vi "Forward Kinematics.vi"(0 "theta":dbl[](array[numeric])=[0.0, 0.0, 0.0] format="%#_15g", 1 "v1d":dbl[](array[numeric]), 2 "v2d":dbl[](array[numeric]), 3 "v3d":dbl[](array[numeric]), 5 "alpha1":dbl=1.5707963267948966, 7 "alpha2":dbl=1.5707963267948966, 9 "beta1":dbl=0.816496580927726, 11 "gamma2":dbl=1.2566370614359172) -> (4 "v1":dbl[](array[numeric]), 6 "v2":dbl[](array[numeric]), 8 "v3":dbl[](array[numeric]), 10 "error?":bool=TRUE, 15 "message":string="Error -23024 occurred at an unidentified location\r\n\r\nPossible reason(s):\n\r\nAnalysis:  No root found.")   [LabVIEW 2017]
uses:
  <vilib>/Utility/error.llb/DialogType.ctl
  <vilib>/Analysis/_algsub.llb/Real Vector Norm.vi
  <vilib>/gmath/zero.llb/nD Nonlinear System Single Solution (Formula).vi
  <vilib>/gmath/NI_Gmath.lvlib
  <vilib>/Analysis/NI_AALPro.lvlib
panel:
  out "beta2":dbl=0.7460127831658564
  out "F(X)":string[](array[string])=["a*d + b*e + c*f - cos(1.256637)", "d*g + e*h + f*i - cos(1.256637)", "g*a + h*b + i*c - cos(1.256637)", "(1.000000)*a + (-0.000000)*b + (-0.000000)*c - cos(1.570796)", "(-0.500000)*d + (0.866025)*e + (-0.000000)*f - cos(1.570796)", "(-0.500000)*g + (-0.866025)*h + (-0.000000)*i - cos(1.570796)", "a^2 + b^2 + c^2 - 1", "d^2 + e^2 + f^2 - 1", "g^2 + h^2 + i^2 - 1"]
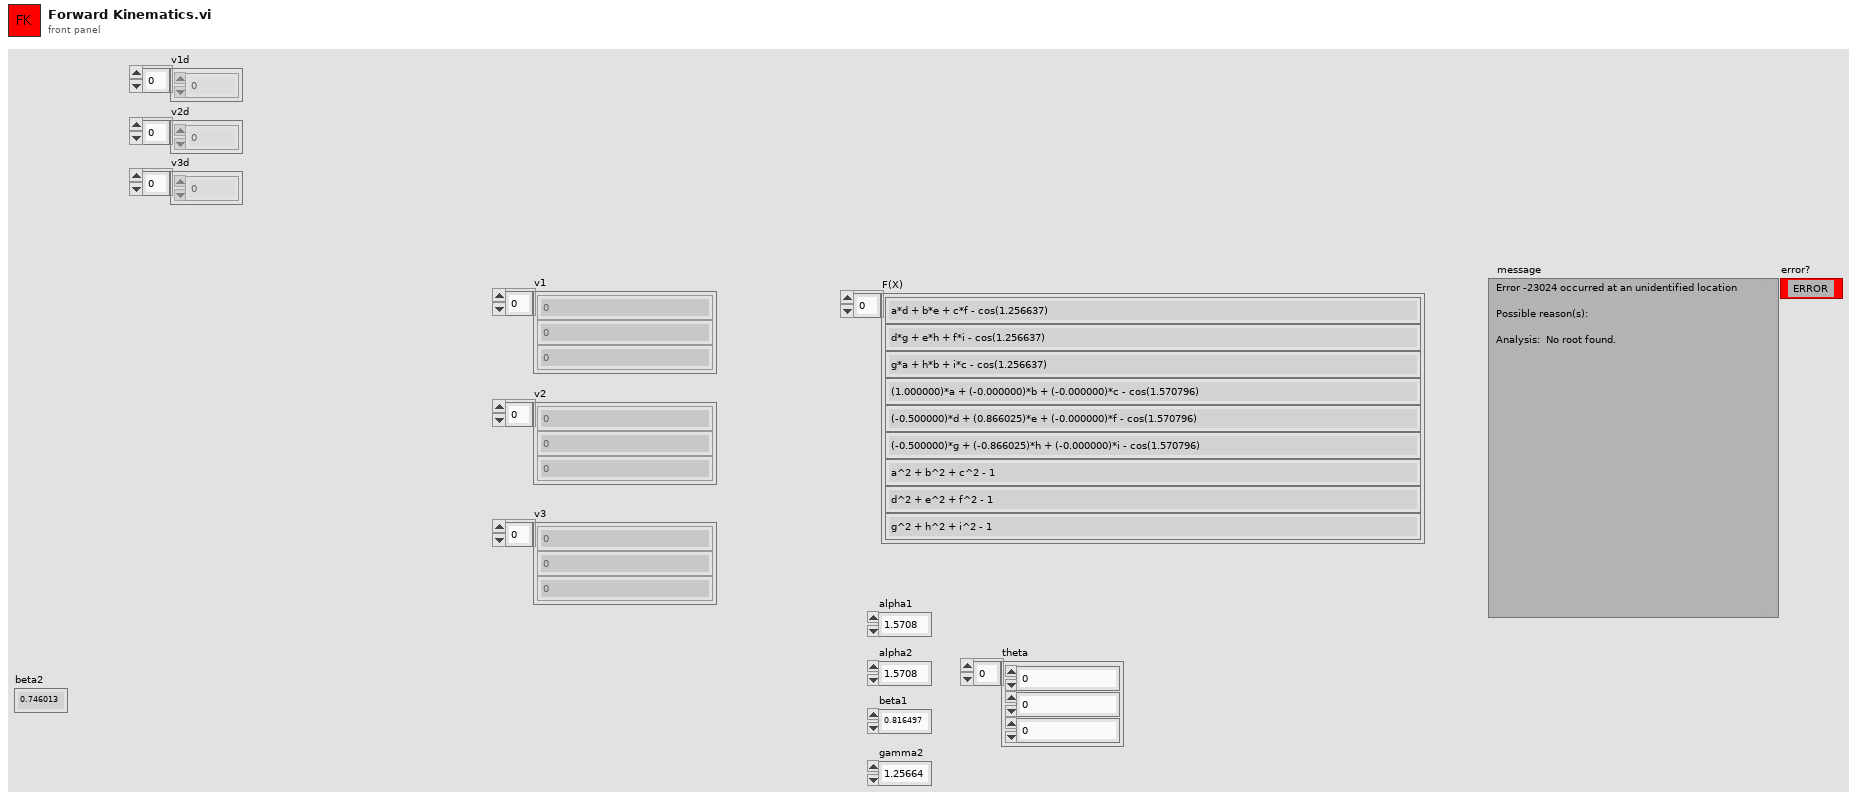
[diagram p1: front panel]
types:
  T1 = typedef "DialogType.ctl" = u16
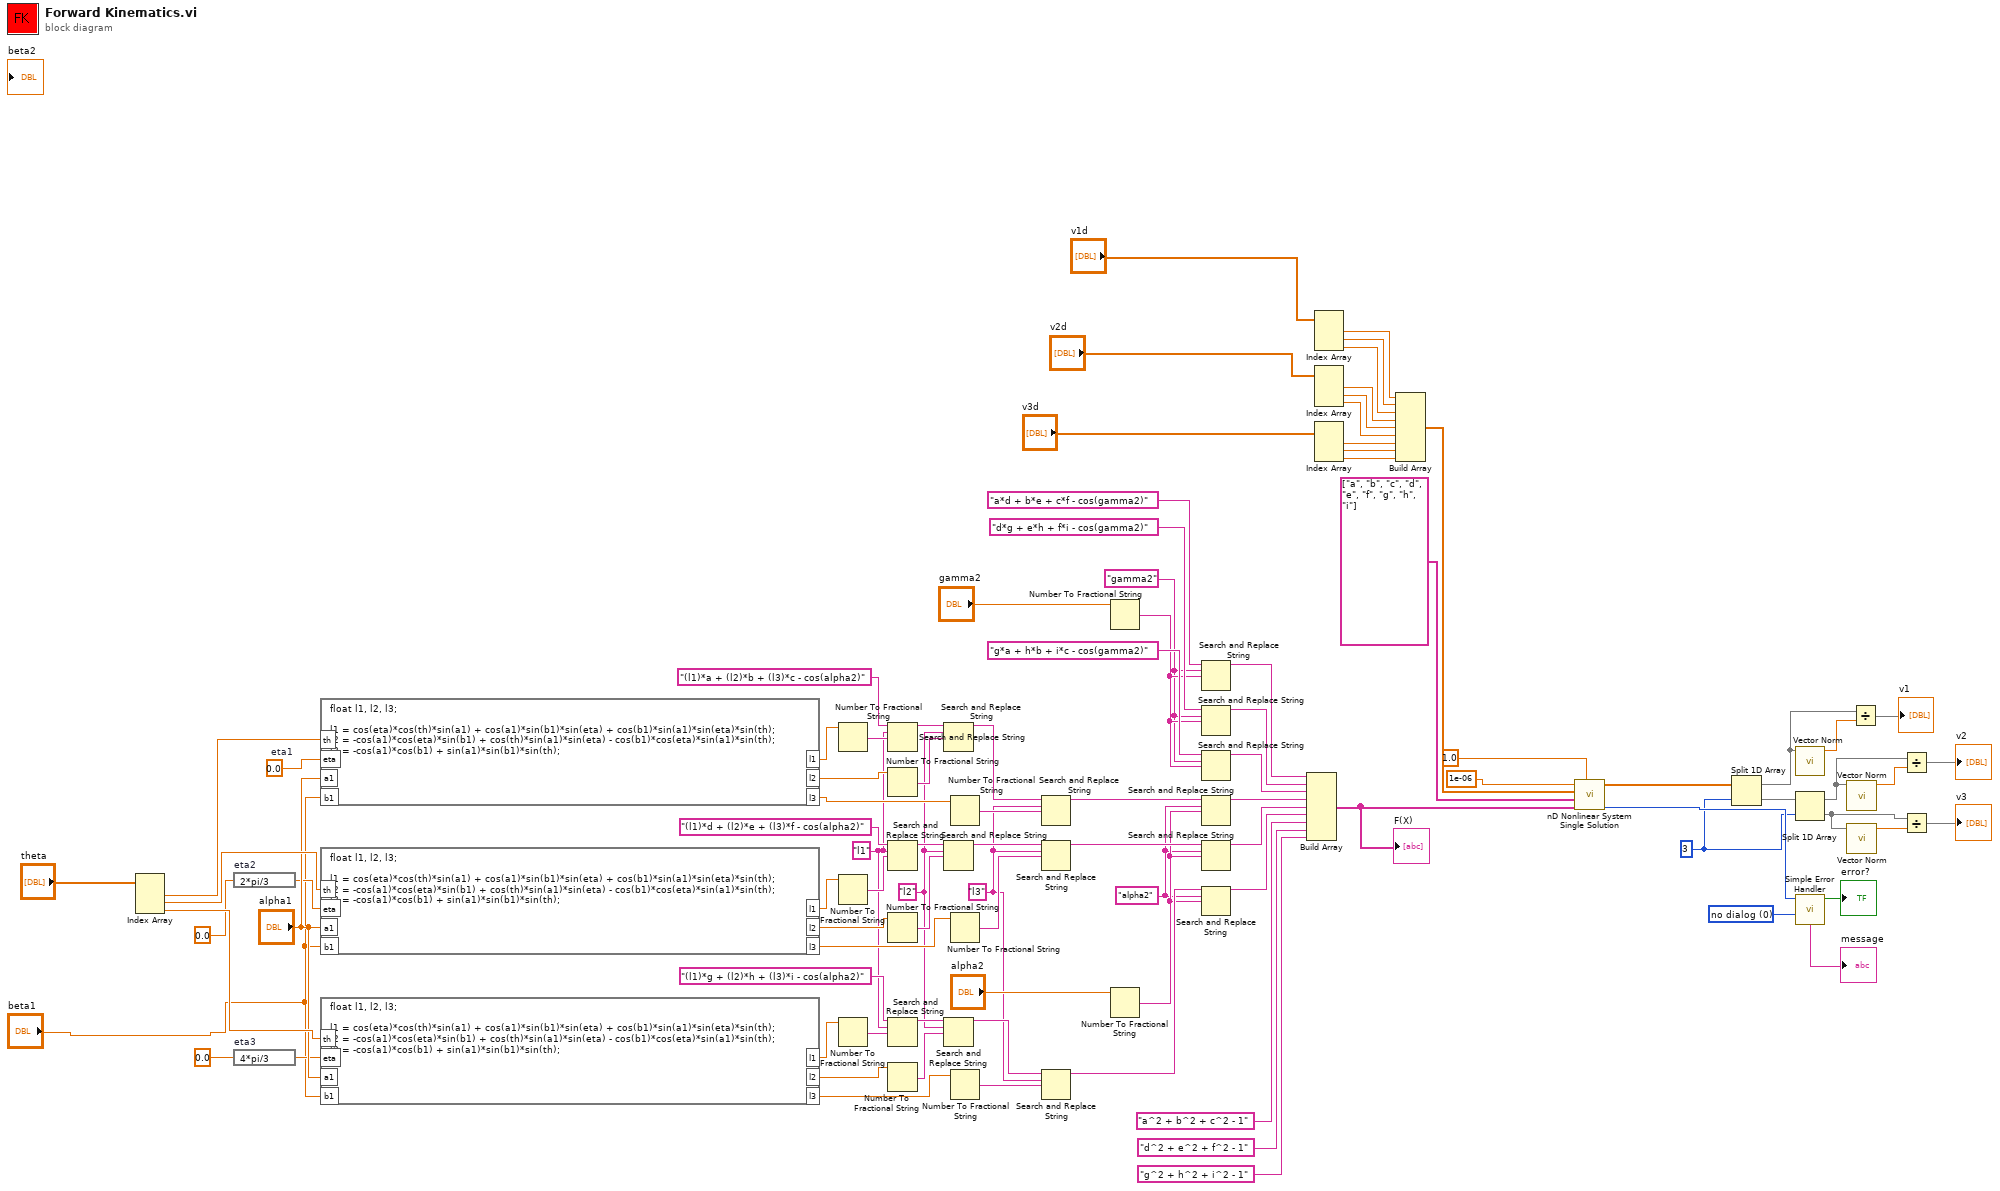
[diagram p0: block diagram]
diagram:
  w21 = 3 ("index")
  w26 = T1 0 items=["no dialog", "OK message", "continue or stop message", "OK message + warnings", "continue/stop + warnings"] ("type of dialog (OK msg:1)")
  w40 = "alpha2" ("search string")
  w41 = "l3" ("search string")
  w42 = "l2" ("search string")
  w43 = "l1" ("search string")
  w39 = "gamma2" ("replace string (\"\")")
  w93 = 0.0  # eta1
  n1 = Index Array(array="theta") -> (element #1=w94:dbl, element #2=w61:dbl, element #3=w60:dbl)  [unwired: 3 in]
  n2 = expression code="2*pi/3" "eta2"(0.0) -> (w52:dbl)
  n3 = expression code="4*pi/3" "eta3"(0.0) -> (w50:dbl)
  n4 = formula code="float l1, l2, l3;\n\nl1 = cos(eta)*cos(th)*sin(a1) + cos(a1)*sin(b1)*sin(eta) + cos(b1)*sin(a1)*sin(eta)*sin(th);\nl2 = -cos(a1)*cos(eta)*sin(b1) + cos(th)*sin(a1)*sin(eta) - cos(b1)*cos(eta)*sin(a1)*sin(th);\nl3 = -cos(a1)*cos(b1) + sin(a1)*sin(b1)*sin(th);"("th"=w94, "eta"=w93, "a1"="alpha1", "b1"="beta1") -> ("l1"=w87:dbl, "l2"=w83:dbl, "l3"=w81:dbl)
  n5 = formula code="float l1, l2, l3;\n\nl1 = cos(eta)*cos(th)*sin(a1) + cos(a1)*sin(b1)*sin(eta) + cos(b1)*sin(a1)*sin(eta)*sin(th);\nl2 = -cos(a1)*cos(eta)*sin(b1) + cos(th)*sin(a1)*sin(eta) - cos(b1)*cos(eta)*sin(a1)*sin(th);\nl3 = -cos(a1)*cos(b1) + sin(a1)*sin(b1)*sin(th);"("th"=w61, "eta"=w52, "a1"="alpha1", "b1"="beta1") -> ("l1"=w72:dbl, "l2"=w76:dbl, "l3"=w78:dbl)
  n6 = formula code="float l1, l2, l3;\n\nl1 = cos(eta)*cos(th)*sin(a1) + cos(a1)*sin(b1)*sin(eta) + cos(b1)*sin(a1)*sin(eta)*sin(th);\nl2 = -cos(a1)*cos(eta)*sin(b1) + cos(th)*sin(a1)*sin(eta) - cos(b1)*cos(eta)*sin(a1)*sin(th);\nl3 = -cos(a1)*cos(b1) + sin(a1)*sin(b1)*sin(th);"("th"=w60, "eta"=w50, "a1"="alpha1", "b1"="beta1") -> ("l1"=w69:dbl, "l2"=w65:dbl, "l3"=w63:dbl)
  n7 = Number To Fractional String(number=w87) -> (F-format string=w86:string)  [unwired: 3 in]
  n8 = Number To Fractional String(number=w72) -> (F-format string=w73:string)  [unwired: 3 in]
  n9 = Number To Fractional String(number=w69) -> (F-format string=w68:string)  [unwired: 3 in]
  n10 = Search and Replace String(input string="(l1)*a + (l2)*b + (l3)*c - cos(alpha2)", search string=w43, replace string=w86) -> (result string=w85:string)  [unwired: 5 in, 3 out]
  n11 = Number To Fractional String(number=w83) -> (F-format string=w82:string)  [unwired: 3 in]
  n12 = Search and Replace String(input string="(l1)*d + (l2)*e + (l3)*f - cos(alpha2)", search string=w43, replace string=w73) -> (result string=w74:string)  [unwired: 5 in, 3 out]
  n13 = Number To Fractional String(number=w76) -> (F-format string=w77:string)  [unwired: 3 in]
  n14 = Search and Replace String(input string="(l1)*g + (l2)*h + (l3)*i - cos(alpha2)", search string=w43, replace string=w68) -> (result string=w67:string)  [unwired: 5 in, 3 out]
  n15 = Number To Fractional String(number=w65) -> (F-format string=w64:string)  [unwired: 3 in]
  n16 = Search and Replace String(input string=w85, search string=w42, replace string=w82) -> (result string=w84:string)  [unwired: 5 in, 3 out]
  n17 = Search and Replace String(input string=w74, search string=w42, replace string=w77) -> (result string=w75:string)  [unwired: 5 in, 3 out]
  n18 = Search and Replace String(input string=w67, search string=w42, replace string=w64) -> (result string=w66:string)  [unwired: 5 in, 3 out]
  n19 = Number To Fractional String(number=w81) -> (F-format string=w80:string)  [unwired: 3 in]
  n20 = Number To Fractional String(number=w78) -> (F-format string=w79:string)  [unwired: 3 in]
  n21 = Number To Fractional String(number=w63) -> (F-format string=w62:string)  [unwired: 3 in]
  n22 = Search and Replace String(input string=w84, search string=w41, replace string=w80) -> (result string=w58:string)  [unwired: 5 in, 3 out]
  n23 = Search and Replace String(input string=w75, search string=w41, replace string=w79) -> (result string=w57:string)  [unwired: 5 in, 3 out]
  n24 = Search and Replace String(input string=w66, search string=w41, replace string=w62) -> (result string=w56:string)  [unwired: 5 in, 3 out]
  n25 = Number To Fractional String(number="gamma2") -> (F-format string=w89:string)  [unwired: 3 in]
  n26 = Number To Fractional String(number="alpha2") -> (F-format string=w55:string)  [unwired: 3 in]
  n27 = Search and Replace String(input string="a*d + b*e + c*f - cos(gamma2)", search string=w39, replace string=w89) -> (result string=w49:string)  [unwired: 5 in, 3 out]
  n28 = Search and Replace String(input string="d*g + e*h + f*i - cos(gamma2)", search string=w39, replace string=w89) -> (result string=w48:string)  [unwired: 5 in, 3 out]
  n29 = Search and Replace String(input string="g*a + h*b + i*c - cos(gamma2)", search string=w39, replace string=w89) -> (result string=w47:string)  [unwired: 5 in, 3 out]
  n30 = Search and Replace String(input string=w58, search string=w40, replace string=w55) -> (result string=w46:string)  [unwired: 5 in, 3 out]
  n31 = Search and Replace String(input string=w57, search string=w40, replace string=w55) -> (result string=w45:string)  [unwired: 5 in, 3 out]
  n32 = Search and Replace String(input string=w56, search string=w40, replace string=w55) -> (result string=w44:string)  [unwired: 5 in, 3 out]
  n33 = Build Array(w49, w48, w47, w46, w45, w44, "a^2 + b^2 + c^2 - 1" ("element"), "d^2 + e^2 + f^2 - 1" ("element"), "g^2 + h^2 + i^2 - 1" ("element")) -> (w37:string[])
  "F(X)" <- w37
  n34 = Index Array(array="v1d") -> (element #1=w36:dbl, element #2=w35:dbl, element #3=w34:dbl)  [unwired: 3 in]
  n35 = Index Array(array="v2d") -> (element #1=w33:dbl, element #2=w32:dbl, element #3=w31:dbl)  [unwired: 3 in]
  n36 = Index Array(array="v3d") -> (element #1=w3:dbl, element #2=w2:dbl, element #3=w1:dbl)  [unwired: 3 in]
  n37 = Build Array(w36, w35, w34, w33, w32, w31, w3, w2, w1) -> (w23:dbl[])
  n38 = call-poly <vilib>:"nD Nonlinear System Single Solution.vi"("accuracy"=1.0, "F(X)"=w37, "X"=string[] ["a", "b", "c", "d", "e", "f", "g", "h", "i"], "Start"=w23, "h"=1e-06) -> ("error"=w27:i32, "Zeroes"=w22:dbl[])  [unwired: 3 in, 2 out]
  n39 = Split 1D Array(array=w22, index=w21) -> (first subarray=w17:dbl[], second subarray=w20:dbl[])
  n40 = call-poly <vilib>:"Vector Norm.vi"("Input Vector"=w17) -> ("norm"=w18:dbl)  [unwired: 9 in, 1 out]
  n41 = Split 1D Array(array=w20, index=w21) -> (first subarray=w15:dbl[], second subarray=w14:dbl[])
  n42 = call <vilib>:"Simple Error Handler.vi"("error code (no error:0)"=w27, "type of dialog (OK msg:1)"=w26) -> ("error?"=→"error?":bool, "message"=→"message":string)  [unwired: 3 in, 3 out]
  n43 = call-poly <vilib>:"Vector Norm.vi"("Input Vector"=w15) -> ("norm"=w16:dbl)  [unwired: 9 in, 1 out]
  n44 = call-poly <vilib>:"Vector Norm.vi"("Input Vector"=w14) -> ("norm"=w13:dbl)  [unwired: 9 in, 1 out]
  n45 = Divide(x=w17, y=w18) -> (x/y=→"v1":dbl[])
  n46 = Divide(x=w15, y=w16) -> (x/y=→"v2":dbl[])
  n47 = Divide(x=w14, y=w13) -> (x/y=→"v3":dbl[])
